vi "Return Add Control Result.vi"(8 "error in (no error)":errorcluster, 10 "GUI Control":refnum<class "GUI Control.lvclass">, 11 "Add Controller (Console2API) in":refnum<class "Console Reply Add Control.lvclass">) -> (0 "error out":errorcluster, 3 "Add Controller (Console2API) out":refnum<class "Console Reply Add Control.lvclass">)   [LabVIEW 2015, in "Console Reply Add Control.lvclass"]
uses:
  Console Reply Add Control.lvclass
  GUI/GUI Controls/GUI Control/GUI Control.lvclass
  Console Reply Add Control.lvclass/Console Reply Add Control.ctl
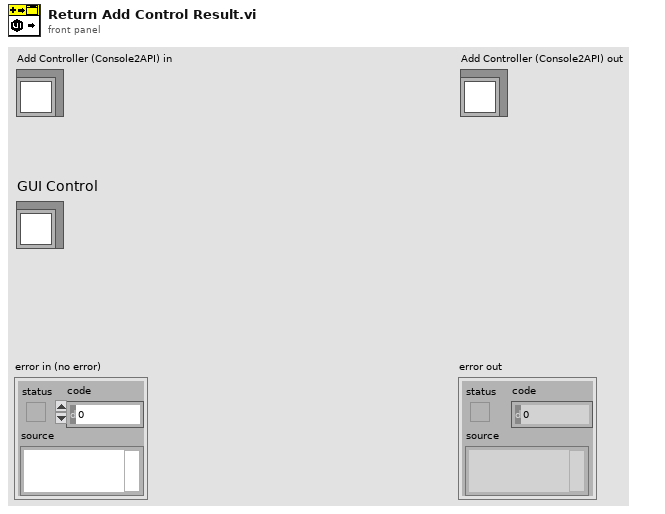
[diagram p1: front panel]
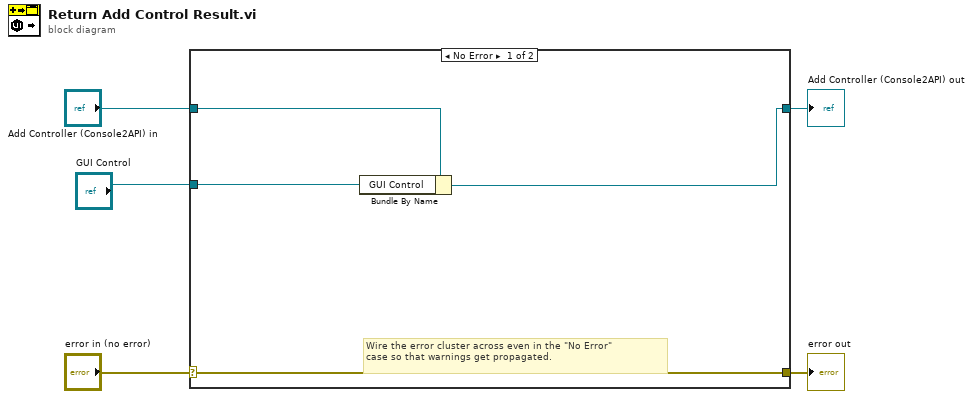
[diagram p0: block diagram]
diagram:
  n1 = case shown="No Error" "error in (no error)" {
    selector: "error in (no error)" -> [w9 w11]
    tunnel: [w9 w11] -> w4
    tunnel: [w7 w10] -> w2
    tunnel: "Add Controller (Console2API) in" -> [w8 w10]
    tunnel: "GUI Control" -> [w6 _]
    frame No Error {
      # "Wire the error cluster across even in the \"No Error\"\ncase so that warnings get propagated."
      n2 = Bundle By Name(cluster=w8, "GUI Control"=w6) -> (w7:refnum<class "Console Reply Add Control.lvclass">)
    }
    frame Error {
    }
  }
  "error out" <- w4
  "Add Controller (Console2API) out" <- w2
